vi "Receive and Display using Event Log.vi"() -> ()   [LabVIEW 2019]
uses:
  <instrlib>/BTICardLib/Public/Controls/Event Log Type.ctl
  <instrlib>/BTICardLib/Private/Initialize By Card Number and Core Number.vi
  <instrlib>/BTICardLib/Private/Configure Core From XML.vi
  <instrlib>/BTI429Lib/Private/Rx/Configure/Configure Rx Channel From XML.vi
  <instrlib>/BTI429Lib/Private/Rx/Configure/Get Rx Label Handle Name.vi
  <instrlib>/BTI429Lib/Private/Core/Action-Status/Start Channel.vi
  <instrlib>/BTI429Lib/Private/Core/Action-Status/Stop Channel.vi
  <instrlib>/BTICardLib/BTICardLV.lvlib
  <instrlib>/BTI429Lib/BTI429LV.lvlib
panel:
  out "core number":i32
  out "channel number":i32
  in  "Channel Configuration XML file name":string="Channel Config.xml"
  in  "Core Configuration XML file name":string="Core Config.xml"
  out "error out":errorcluster
  in  "Card Number":i32
  out "Data 2":u32 format="%x"
  out "Data 1":u32 format="%x"
  out "Default":u32 format="%x"
  in  "stop":bool
  # "ARINC 429: Receive Labels"
  # "©2016 Astronics Ballard Technology"
  # "This program opens the specified card, and configures the receive channel to\nreceive 2 GPS messages into separate Message Records, and receive all other\nmessages into a default Message Record. The GPS message labels are read from\nthe Channel Configuration XML file.\n\nThe label definitions enable Event Log Recording of Message actitivty. The \nEvent Log is polled for 429 Messages and when a specific label has been \nreceived, its data is updated on the front panel."
  # "Always Stop the card\nand Close the card when\ndone. Otherwise, the hardware\ncontinues to operate."
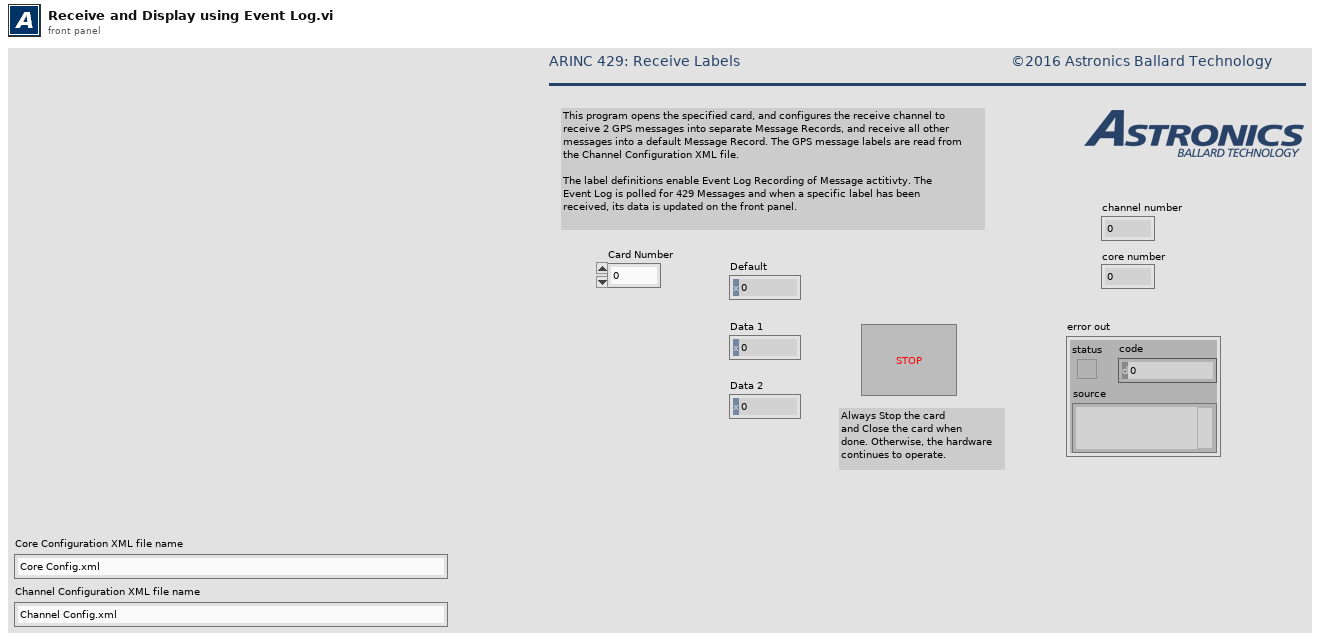
[diagram p1: front panel]
types:
  T1 = typedef "BTICardLV.lvlib/Event Log Type.ctl" = u32
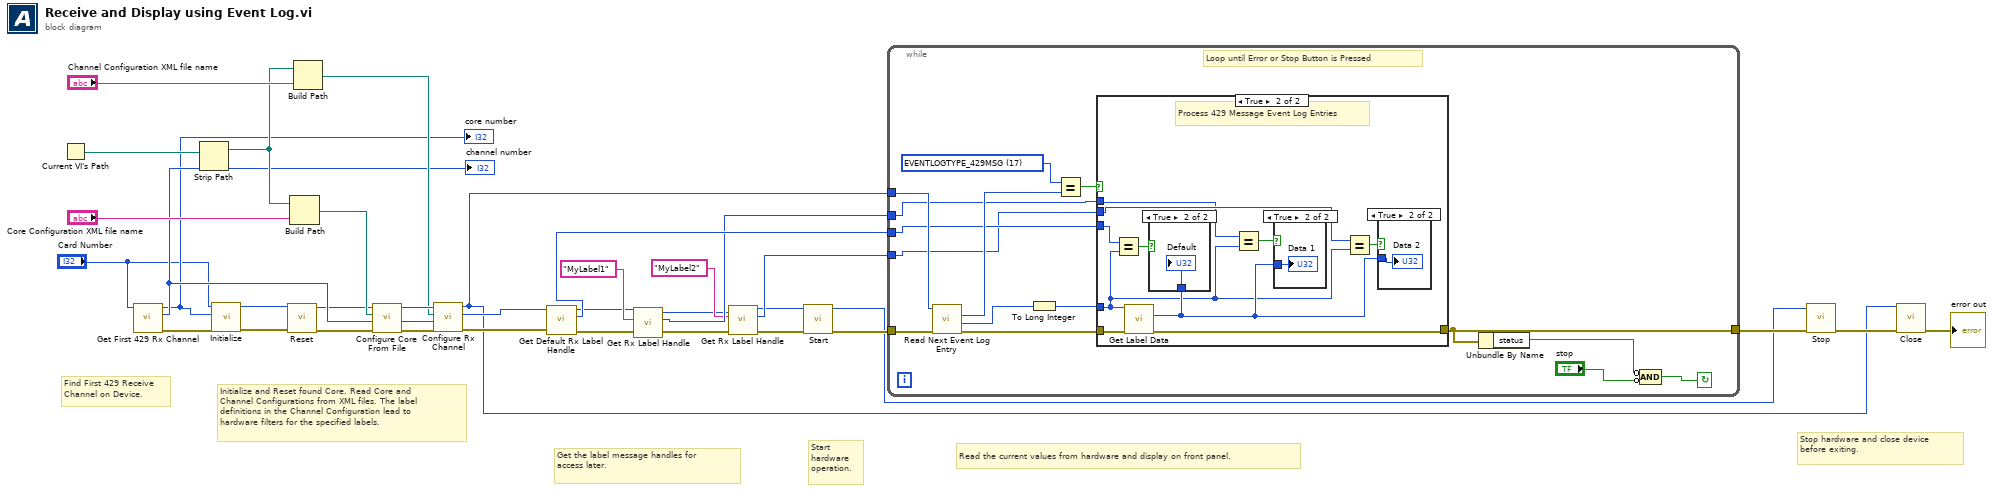
[diagram p0: block diagram]
diagram:
  # "Stop hardware and close device\nbefore exiting."
  # "Read the current values from hardware and display on front panel."
  # "Start\nhardware\noperation."
  # "Get the label message handles for\naccess later."
  # "Initialize and Reset found Core. Read Core and\nChannel Configurations from XML files. The label\ndefinitions in the Channel Configuration lead to\nhardware filters for the specified labels."
  # "Find First 429 Receive\nChannel on Device."
  n1 = Current VI's Path() -> (path=w14:path)
  n2 = call "Get First 429 Rx Channel.vi"("Card Number"="Card Number") -> ("error out"=w8:errorcluster, "Channel Number"=w7:i32, "Core Number"=w6:i32)  [unwired: 8 in]
  "channel number" <- w7
  "core number" <- w6
  n3 = Strip Path(path=w14) -> (stripped path=w12:path)  [unwired: 1 out]
  n4 = call-poly <instrlib>:"Initialize.vi"("error in (no error)"=w8, "core number"=w6, "card number"="Card Number") -> ("error out"=w4:errorcluster, "core handle out"=w2:u64)  [unwired: 7 in]
  n5 = call <instrlib>:"Reset.vi"("error in (no error)"=w4, "core handle in"=w2) -> ("error out"=w3:errorcluster, "core handle out"=w1:u64)  [unwired: 8 in]
  n6 = Build Path(base path=w12, name or relative path="Core Configuration XML file name") -> (appended path=w10:path)
  n7 = Build Path(base path=w12, name or relative path="Channel Configuration XML file name") -> (appended path=w9:path)
  n8 = call-poly <instrlib>:"Configure Core From File.vi"("error in (no error)"=w3, "configuration file path"=w10, "core handle in"=w1) -> ("error out"=w26:errorcluster, "core handle out"=w21:u64)  [unwired: 7 in]
  n9 = call-poly <instrlib>:"Configure Rx Channel.vi"("error in (no error)"=w26, "channel number in"=w7, "configuration file path"=w9, "core handle in"=w21) -> ("error out"=w35:errorcluster, "channel handle out"=w20:u64, "core handle out"=w19:u64)  [unwired: 5 in]
  n10 = call <instrlib>:"Get Default Rx Label Handle.vi"("error in (no error)"=w35, "channel handle in"=w20) -> ("error out"=w34:errorcluster, "default label handle out"=w30:u64, "channel handle out"=w18:u64)  [unwired: 7 in]
  n11 = call-poly <instrlib>:"Get Rx Label Handle.vi"("error in (no error)"=w34, "label name"="MyLabel1", "channel handle in"=w18) -> ("error out"=w33:errorcluster, "label handle out"=w29:u64, "channel handle out"=w17:u64)  [unwired: 6 in]
  n12 = call-poly <instrlib>:"Get Rx Label Handle.vi"("error in (no error)"=w33, "label name"="MyLabel2", "channel handle in"=w17) -> ("error out"=w32:errorcluster, "label handle out"=w28:u64, "channel handle out"=w16:u64)  [unwired: 6 in]
  n13 = call-poly <instrlib>:"Start.vi"("error in (no error)"=w32, "channel handle in"=w16) -> ("error out"=w31:errorcluster, "channel handle out"=w15:u64)  [unwired: 8 in]
  n14 = while {
    tunnel: w31 -> [w47]
    tunnel: w30 -> [w41]
    tunnel: w29 -> [w38]
    tunnel: w28 -> [w39]
    tunnel: [w40] -> w22
    tunnel: w19 -> [w45]
    stop <- w50 continue-if-true
    w43 = T1 17 items=["EVENTLOGTYPE_NONE"=0, "EVENTLOGTYPE_1553MSG"=1, "EVENTLOGTYPE_1553OPCODE"=2, "EVENTLOGTYPE_1553HALT"=3, "EVENTLOGTYPE_1553PAUSE"=4, "EVENTLOGTYPE_1553LIST"=5, "EVENTLOGTYPE_1553SERIAL"=6, "EVENTLOGTYPE_429MSG"=17, "EVENTLOGTYPE_429OPCODE"=18, "EVENTLOGTYPE_429HALT"=19, "EVENTLOGTYPE_429PAUSE"=20, "EVENTLOGTYPE_429LIST"=21, "EVENTLOGTYPE_429ERR"=22, "EVENTLOGTYPE_DIOEDGE"=96, "EVENTLOGTYPE_DIOFAULT"=97, "EVENTLOGTYPE_BITERROR"=113] ("x")
    # "Loop until Error or Stop Button is Pressed"
    n15 = call <instrlib>:"Read Next Event Log Entry.vi"("error in (no error)"=w47, "core handle in"=w45) -> ("error out"=w46:errorcluster, "info tag"=w36:u64, "event log entry type"=w44:T1)  [unwired: 4 in, 3 out]
    n16 = To Long Integer(number=w36) -> (32bit integer=w37:i32)
    n17 = Equal?(x=w43, y=w44) -> (x = y?=w42:bool)
    n18 = case shown="True" w42 {
      tunnel: w46 -> [w51 w61]
      tunnel: w37 -> [_ w53]
      tunnel: w41 -> [_ w58]
      tunnel: [w51 w57] -> w40
      tunnel: w39 -> [_ w55]
      tunnel: w38 -> [_ w52]
      frame False {
        # "No 429 Messages to Process"
      }
      frame True {
        # "Process 429 Message Event Log Entries"
        n19 = Equal?(x=w58, y=w53) -> (x = y?=w59:bool)
        n20 = call <instrlib>:"Get Label Data.vi"("error in (no error)"=w61, "label handle in"=w53) -> ("error out"=w57:errorcluster, "value"=w60:u32)  [unwired: 7 in, 1 out]
        n21 = case shown="True" w59 {
          tunnel: w60 -> [_ w62]
          frame False {
          }
          frame True {
            "Default" <- w62
          }
        }
        n22 = Equal?(x=w52, y=w53) -> (x = y?=w54:bool)
        n23 = case shown="True" w54 {
          tunnel: w60 -> [_ w63]
          frame False {
          }
          frame True {
            "Data 1" <- w63
          }
        }
        n24 = Equal?(x=w55, y=w53) -> (x = y?=w56:bool)
        n25 = case shown="True" w56 {
          tunnel: w60 -> [_ w64]
          frame False {
          }
          frame True {
            "Data 2" <- w64
          }
        }
      }
    }
    n26 = Unbundle By Name(w40) -> ("status"=w48:bool)
    n27 = Compound Arithmetic op=AND(invert w48, invert "stop") -> (w50:bool)
  }
  n28 = call-poly <instrlib>:"Stop.vi"("error in (no error)"=w22, "channel handle in"=w15) -> ("error out"=w27:errorcluster)  [unwired: 8 in, 1 out]
  n29 = call <instrlib>:"Close.vi"("error in (no error)"=w27, "core handle in"=w19) -> ("error out"=→"error out":errorcluster)  [unwired: 8 in, 1 out]
